vi "Check for DAQmx Errors.vi"(7 "USB Camera in":refnum<class "USB Camera.lvclass">, 8 "error in (no error)":errorcluster, 9 "DAQmx Switch in":refnum<class "DAQmx Switch.lvclass">, 10 "DAQmx Servo in":refnum<class "DAQmx Servo.lvclass">, 11 "DAQmx Force Sensor in":refnum<class "DAQmx Force Sensor.lvclass">) -> (0 "error out":errorcluster, 1 "DAQmx Switch out":refnum<class "DAQmx Switch.lvclass">, 2 "DAQmx Servo out":refnum<class "DAQmx Servo.lvclass">, 3 "DAQmx Force Sensor out":refnum<class "DAQmx Force Sensor.lvclass">, 5 "USB Camera out":refnum<class "USB Camera.lvclass">)   [LabVIEW 2020]
uses:
  Actuators/Switches/DAQmx Switch/DAQmx Switch.lvclass
  C:/Users/Haslach/Documents/Inflation-Apparatus/src/Hardware/General Hardware.lvclass
  Sensors/Cameras/USB Camera/USB Camera.lvclass
  Sensors/Force Sensors/DAQmx Force Sensor/DAQmx Force Sensor.lvclass
  Actuators/Servos/DAQmx Servo/DAQmx Servo.lvclass
  General Hardware.lvclass
  C:/Users/Haslach/Documents/Inflation-Apparatus/src/Hardware/Sensors/Cameras/Camera.lvclass
  C:/Users/Haslach/Documents/Inflation-Apparatus/src/Hardware/Sensors/Sensor.lvclass
  C:/Users/Haslach/Documents/Inflation-Apparatus/src/Hardware/Sensors/Cameras/USB Camera/USB Camera.lvclass
  C:/Users/Haslach/Documents/Inflation-Apparatus/src/Hardware/Sensors/Force Sensors/Force Sensor.lvclass
  C:/Users/Haslach/Documents/Inflation-Apparatus/src/Hardware/Sensors/Force Sensors/DAQmx Force Sensor/DAQmx Force Sensor.lvclass
  C:/Users/Haslach/Documents/Inflation-Apparatus/src/Hardware/Actuators/Servos/Servo.lvclass
  C:/Users/Haslach/Documents/Inflation-Apparatus/src/Hardware/Actuators/Actuator.lvclass
  C:/Users/Haslach/Documents/Inflation-Apparatus/src/Hardware/Actuators/Servos/DAQmx Servo/DAQmx Servo.lvclass
  C:/Users/Haslach/Documents/Inflation-Apparatus/src/Hardware/Actuators/Switches/Switch.lvclass
  C:/Users/Haslach/Documents/Inflation-Apparatus/src/Hardware/Actuators/Switches/DAQmx Switch/DAQmx Switch.lvclass
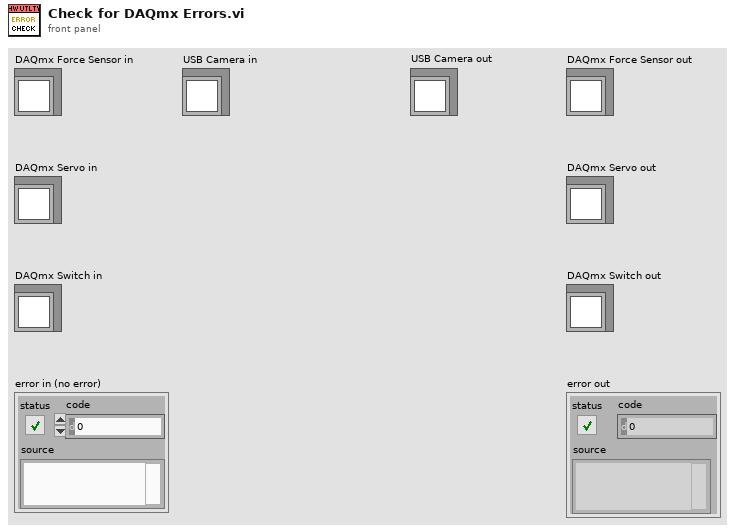
[diagram p1: front panel]
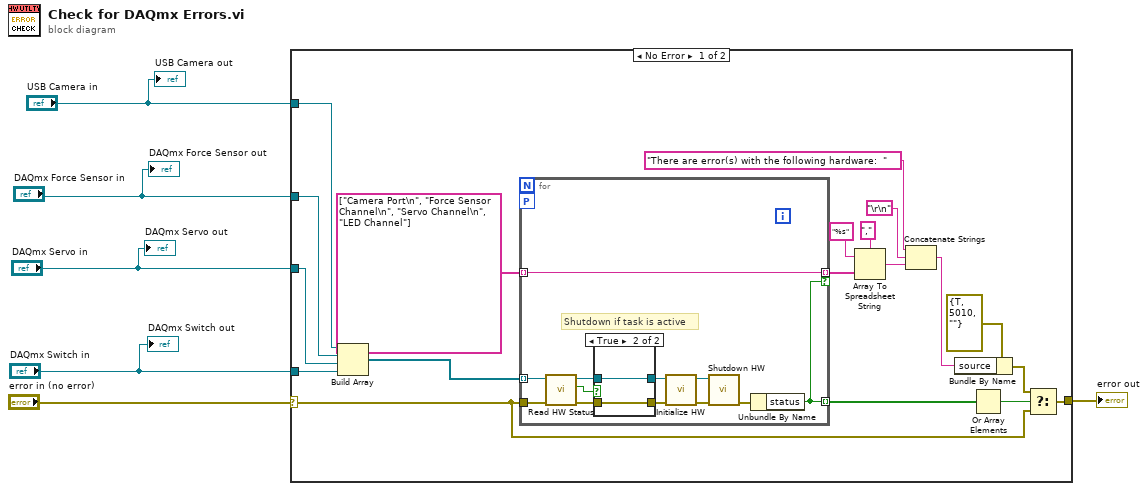
[diagram p0: block diagram]
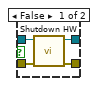
[diagram p2: hidden frame]
diagram:
  n1 = case shown="No Error" "error in (no error)" {
    selector: "error in (no error)" -> [w14 w44]
    tunnel: "USB Camera in" -> [w22 _]
    tunnel: "DAQmx Force Sensor in" -> [w23 _]
    tunnel: "DAQmx Switch in" -> [w25 _]
    tunnel: "DAQmx Servo in" -> [w24 _]
    tunnel: [w17 w44] -> w1
    frame No Error {
      n2 = Build Array(w22, w23, w24, w25) -> (w20:refnum<class "General Hardware.lvclass">[])
      n3 = for {
        tunnel: w14 -> [w29]
        tunnel: string[] ["Camera Port\n", "Force Sensor Channel\n", "Servo Channel\n", "LED Channel"] -> [w34] mode=indexing
        tunnel: [w34] -> w13 mode=indexing if=w31
        tunnel: w20 -> [w30] mode=indexing
        tunnel: [w31] -> w19 mode=indexing
        workers-P: _ -> [_]
        # "Shutdown if task is active"
        n4 = call "Read HW Status.vi"("error in (no error)"=w29, "General Hardware in"=w30) -> ("error out"=w28:errorcluster, "shutdown?"=w26:bool, "General Hardware out"=w27:refnum<class "General Hardware.lvclass">)  [unwired: 7 in]
        n5 = case shown="True" w26 {
          tunnel: [w41 w43] -> w33
          tunnel: [w40 w42] -> w32
          tunnel: w28 -> [w39 w42]
          tunnel: w27 -> [w38 w43]
          frame False {
            n6 = call-dynamic "Shutdown HW.vi"("error in (no error)"=w39, "General Hardware in"=w38) -> ("error out"=w40:errorcluster, "General Hardware out"=w41:refnum<class "General Hardware.lvclass">)  [unwired: 8 in]
          }
          frame True {
          }
        }
        n7 = call-dynamic "Initialize HW.vi"("error in (no error)"=w32, "General Hardware in"=w33) -> ("error out"=w37:errorcluster, "General Hardware out"=w36:refnum<class "General Hardware.lvclass">)  [unwired: 8 in]
        n8 = call-dynamic "Shutdown HW.vi"("error in (no error)"=w37, "General Hardware in"=w36) -> ("error out"=w35:errorcluster)  [unwired: 8 in, 1 out]
        n9 = Unbundle By Name(w35) -> ("status"=w31:bool)
      }
      n10 = Array To Spreadsheet String(delimiter (Tab)=",", array=w13, 3:"%s" ("format string")) -> (spreadsheet string=w10:string)
      n11 = Concatenate Strings("There are error(s) with the following hardware:  ", "\r\n", w10) -> (w7:string)
      n12 = Bundle By Name(cluster=errorcluster {"status"=TRUE, "code"=5010, "source"=""} ("error constant"), "source"=w7) -> (w15:errorcluster)
      n13 = Or Array Elements(Boolean array=w19) -> (logical OR=w18:bool)
      n14 = Select(t=w15, s=w18, f=w14) -> (s? t:f=w17:errorcluster)
    }
    frame Error {
    }
  }
  "error out" <- w1
  "DAQmx Switch out" <- "DAQmx Switch in"
  "USB Camera out" <- "USB Camera in"
  "DAQmx Force Sensor out" <- "DAQmx Force Sensor in"
  "DAQmx Servo out" <- "DAQmx Servo in"
